vi "Blocking Performance Test Core.vi"(6 "Packets Sent":refnum<vi>, 8 "error in":errorcluster, 10 "test run":string="fbf_1", 11 "Test Paramaters":T1={"Interference sig. freq."=30, "Wanted Signal"=2426.0, "Blocking Signal"=2426.0, "Measurement res."=10} {"Measurement res." format="%.0f MHz"; "Blocking Signal" format="%#_gdBm"; "Interference sig. freq." format="%.0f MHz"; "Wanted Signal" format="%#_gdBm"}) -> (0 "error out":errorcluster, 1 "PER":dbl, 2 "Results":string, 3 "received Packets":u32)   [LabVIEW 2013]
doc: "This state machine will perform a single test based on a set of paramaters fed into the input and provide a set of results."
uses:
  Test Parameters.ctl
  Main Test Control.ctl
  Sig Gen Control Command.ctl
  Waveform Details Control.ctl
  UUT Control Command.ctl
  Globals/Hardware Configuration Global.vi
  Globals/Test Criteria Global.vi
panel:
  out "Send Packet Count":u32
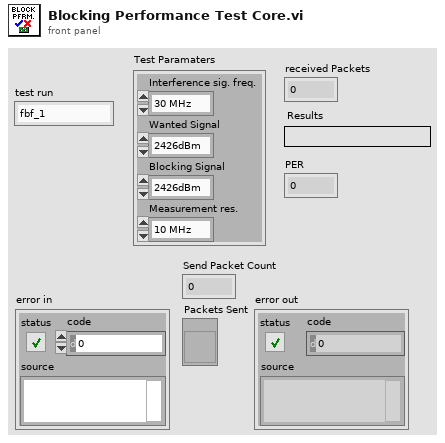
[diagram p1: front panel]
types:
  T1 = typedef "Test Parameters.ctl" = cluster{"Interference sig. freq.":u32, "Wanted Signal":dbl, "Blocking Signal":dbl, "Measurement res.":u32}
  T2 = typedef "Main Test Control.ctl" = enum16{"Initialise", "Stop", "Init WFG 1", "Init WFG 2", "Validate Temperature", "Init UUT", "Begin Test", "Send Packet", "Check Received Packets", "Temerature correction cycle"}
  T3 = typedef "Waveform Details Control.ctl" = cluster{"Power (dB)":dbl, "Frequency (MHz)":u32}
  T4 = typedef "Sig Gen Control Command.ctl" = enum16{"Initialise", "Start", "Stop", "Set Frequency", "Set Power", "Send Packet"}
  T5 = typedef "UUT Control Command.ctl" = enum16{"Initialise packet count", "Read Packet Count", "Return Temperature", "Return Operating Voltage"}
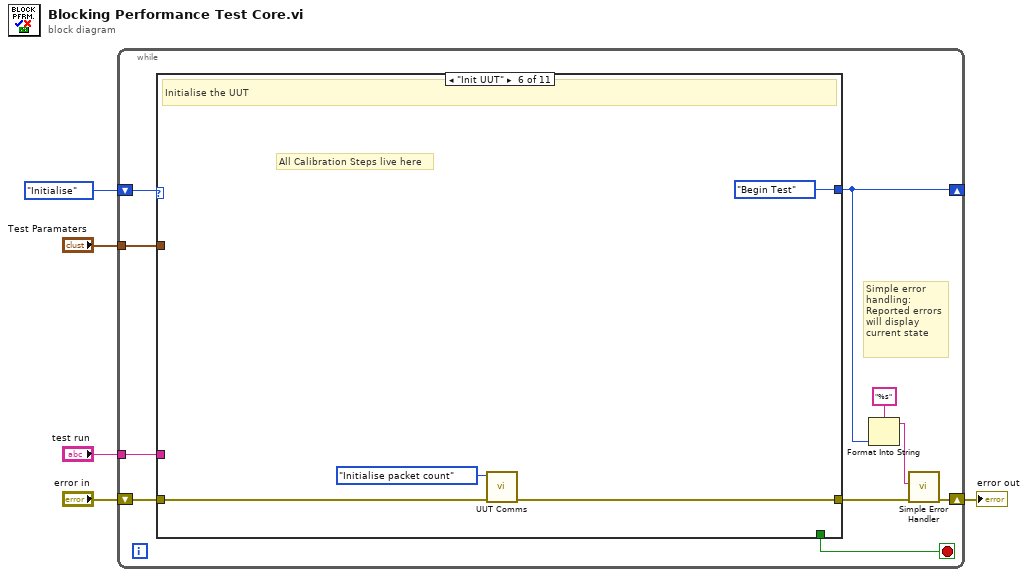
[diagram p0: block diagram]
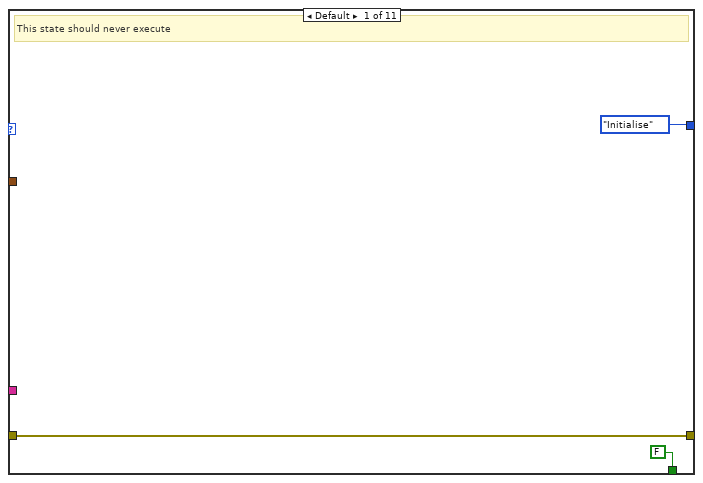
[diagram p2: hidden frame]
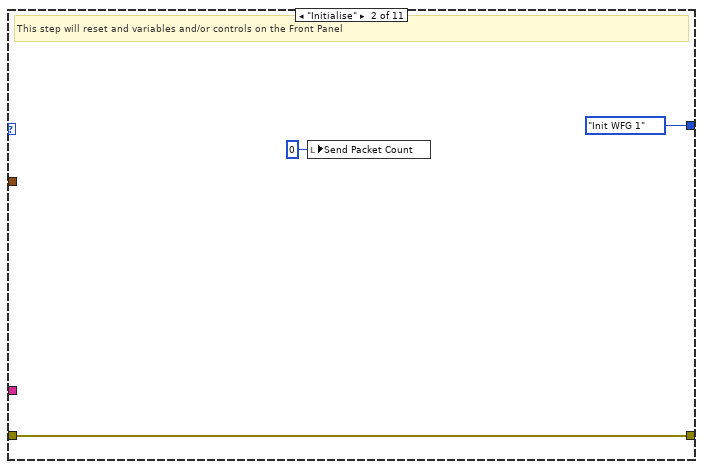
[diagram p3: hidden frame]
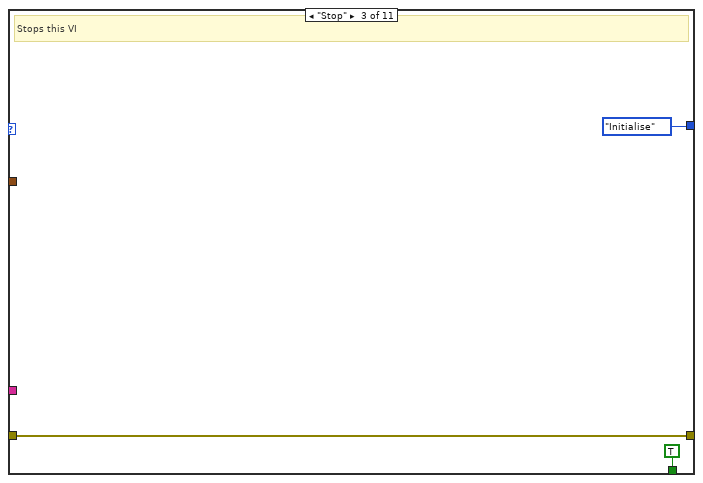
[diagram p4: hidden frame]
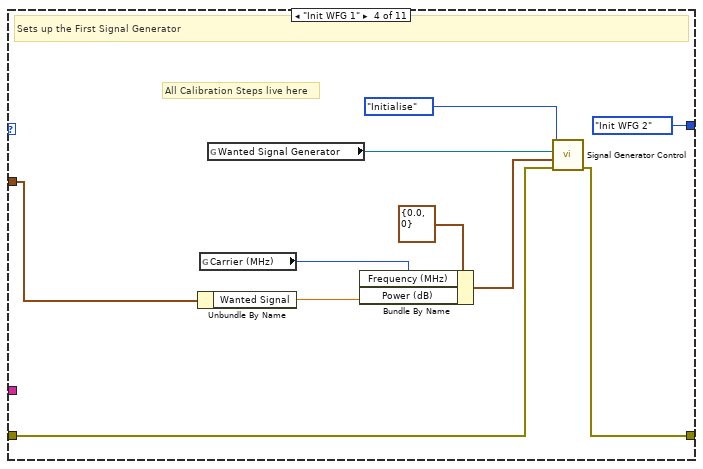
[diagram p5: hidden frame]
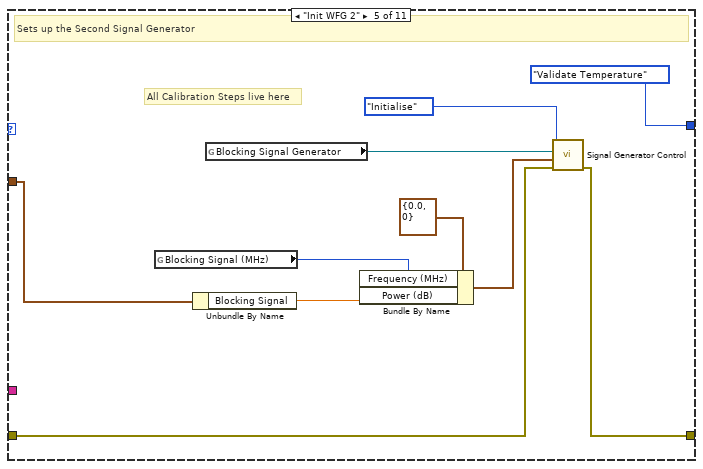
[diagram p6: hidden frame]
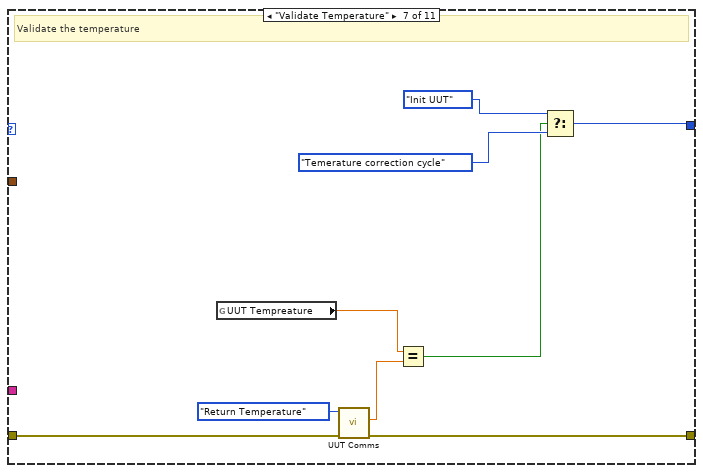
[diagram p7: hidden frame]
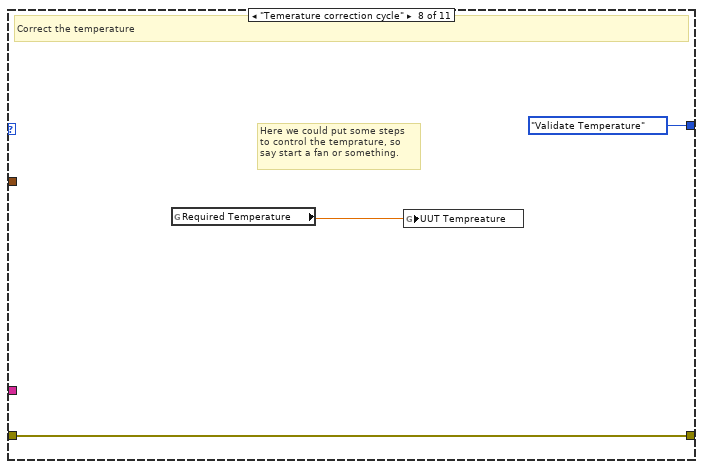
[diagram p8: hidden frame]
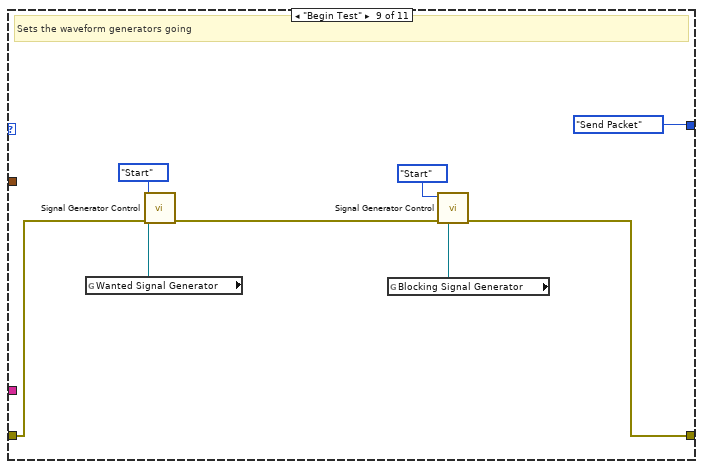
[diagram p9: hidden frame]
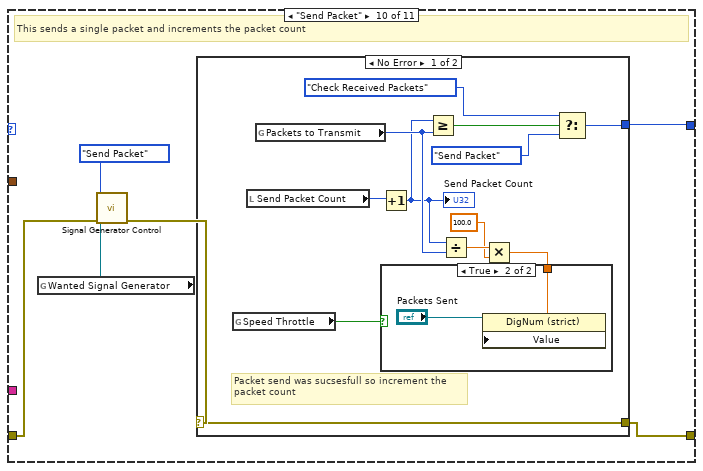
[diagram p10: hidden frame]
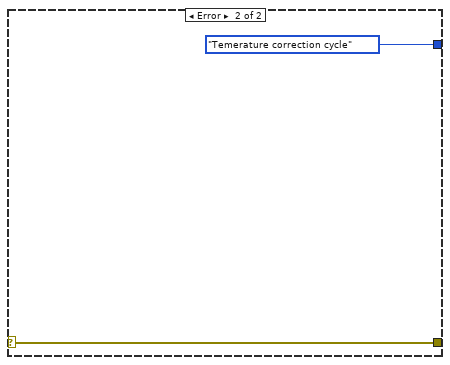
[diagram p12: hidden frame]
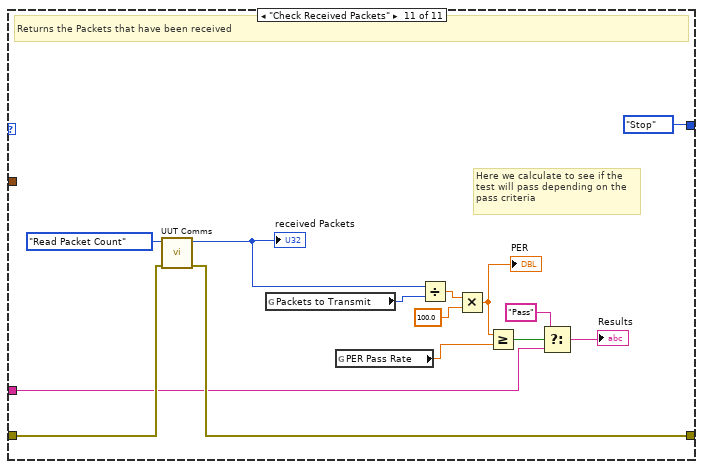
[diagram p13: hidden frame]
diagram:
  n1 = while {
    shift-right: [w10] -> _
    shift-left: Main_Test_Control."Initialise" ("Control") -> [w14]
    shift-right: [w11] -> w3
    shift-left: "error in" -> [w13]
    tunnel: "Test Paramaters" -> [w7]
    tunnel: "test run" -> [w6]
    stop <- w15 stop-if-true
    # "Simple error\nhandling:\nReported errors\nwill display\ncurrent state"
    n2 = case shown="\"Init UUT\"" w14 {
      tunnel: [FALSE _ TRUE _ _ _ _ _ _ _ _] -> w15
      tunnel: [Main_Test_Control."Initialise" ("Control") Main_Test_Control."Init WFG 1" ("Control") Main_Test_Control."Initialise" ("Control") Main_Test_Control."Init WFG 2" ("Control") Main_Test_Control."Validate Temperature" ("Control") Main_Test_Control."Begin Test" ("Control") w52 Main_Test_Control."Validate Temperature" ("Control") Main_Test_Control."Send Packet" ("Control") w69 Main_Test_Control."Stop" ("Control")] -> w10
      tunnel: w13 -> [w16 w19 w22 w29 w39 w48 w57 w59 w63 w72 w103]
      tunnel: [w16 w19 w22 w28 w38 w47 w56 w59 w62 w70 w102] -> w12
      tunnel: w7 -> [_ _ _ w26 w37 _ _ _ _ _ _]
      tunnel: w6 -> [_ _ _ _ _ _ _ _ _ _ w91]
      frame Default {
        # "This state should never execute"
      }
      frame "Initialise" {
        # "This step will reset and variables and/or controls on the Front Panel"
        n3 = local write "Send Packet Count"(u32 0 ("Send Packet Count")) -> ()
      }
      frame "Stop" {
        # "Stops this VI"
      }
      frame "Init WFG 1" {
        # "All Calibration Steps live here"
        # "Sets up the First Signal Generator"
        n4 = Unbundle By Name(w26) -> ("Wanted Signal"=w25:dbl)
        n5 = global read "Test Criteria Global.vi" "Carrier (MHz)"() -> (w27:u32)
        n6 = global read "Hardware Configuration Global.vi" "Wanted Signal Generator"() -> (w33:refnum<k15>)
        n7 = Bundle By Name(cluster=T3 {"Power (dB)"=0.0, "Frequency (MHz)"=0} ("Waveform Data"), "Frequency (MHz)"=w27, "Power (dB)"=w25) -> (w30:T3)
        n8 = call "Signal Generator Control.vi"("error in"=w29, "Waveform Data"=w30, "Device"=w33, "Command"=Sig_Gen_Control_Command."Initialise") -> ("error out"=w28:errorcluster)  [unwired: 6 in, 1 out]
      }
      frame "Init WFG 2" {
        # "All Calibration Steps live here"
        # "Sets up the Second Signal Generator"
        n9 = global read "Test Criteria Global.vi" "Blocking Signal (MHz)"() -> (w35:u32)
        n10 = Unbundle By Name(w37) -> ("Blocking Signal"=w36:dbl)
        n11 = global read "Hardware Configuration Global.vi" "Blocking Signal Generator"() -> (w43:refnum<k15>)
        n12 = Bundle By Name(cluster=T3 {"Power (dB)"=0.0, "Frequency (MHz)"=0} ("Waveform Data"), "Frequency (MHz)"=w35, "Power (dB)"=w36) -> (w40:T3)
        n13 = call "Signal Generator Control.vi"("error in"=w39, "Waveform Data"=w40, "Device"=w43, "Command"=Sig_Gen_Control_Command."Initialise") -> ("error out"=w38:errorcluster)  [unwired: 6 in, 1 out]
      }
      frame "Init UUT" {
        # "All Calibration Steps live here"
        # "Initialise the UUT"
        n14 = call "UUT Comms.vi"("error in"=w48, "Command"=UUT_Control_Command."Initialise packet count") -> ("error out"=w47:errorcluster)  [unwired: 6 in, 3 out]
      }
      frame "Validate Temperature" {
        # "Validate the temperature"
        n15 = global read "Test Criteria Global.vi" "UUT Tempreature"() -> (w51:dbl)
        n16 = call "UUT Comms.vi"("error in"=w57, "Command"=UUT_Control_Command."Return Temperature") -> ("error out"=w56:errorcluster, "Temperature"=w49:dbl)  [unwired: 6 in, 2 out]
        n17 = Equal?(x=w51, y=w49) -> (x = y?=w50:bool)
        n18 = Select(t=Main_Test_Control."Init UUT" ("Control"), s=w50, f=Main_Test_Control."Temerature correction cycle" ("Control")) -> (s? t:f=w52:T2)
      }
      frame "Temerature correction cycle" {
        # "Here we could put some steps\nto control the temprature, so\nsay start a fan or something."
        # "Correct the temperature"
        n19 = global read "Test Criteria Global.vi" "Required Temperature"() -> (w58:dbl)
        n20 = global write "Test Criteria Global.vi" "UUT Tempreature"(w58) -> ()
      }
      frame "Begin Test" {
        # "Sets the waveform generators going"
        n21 = global read "Hardware Configuration Global.vi" "Wanted Signal Generator"() -> (w68:refnum<k15>)
        n22 = call "Signal Generator Control.vi"("error in"=w63, "Device"=w68, "Command"=Sig_Gen_Control_Command."Start") -> ("error out"=w64:errorcluster)  [unwired: 7 in, 1 out]
        n23 = global read "Hardware Configuration Global.vi" "Blocking Signal Generator"() -> (w67:refnum<k15>)
        n24 = call "Signal Generator Control.vi"("error in"=w64, "Device"=w67, "Command"=Sig_Gen_Control_Command."Start") -> ("error out"=w62:errorcluster)  [unwired: 7 in, 1 out]
      }
      frame "Send Packet" {
        # "This sends a single packet and increments the packet count"
        n25 = global read "Hardware Configuration Global.vi" "Wanted Signal Generator"() -> (w74:refnum<k15>)
        n26 = call "Signal Generator Control.vi"("error in"=w72, "Device"=w74, "Command"=Sig_Gen_Control_Command."Send Packet") -> ("error out"=w71:errorcluster)  [unwired: 7 in, 1 out]
        n27 = case shown="No Error" w71 {
          selector: w71 -> [w81 w90]
          tunnel: [w81 w90] -> w70
          tunnel: [w82 Main_Test_Control."Temerature correction cycle" ("Control")] -> w69
          frame No Error {
            # "Packet send was sucsesfull so increment the\npacket count"
            n28 = global read "Test Criteria Global.vi" "Speed Throttle"() -> (w76:bool)
            n29 = local read "Send Packet Count"() -> (w86:u32)
            n30 = global read "Test Criteria Global.vi" "Packets to Transmit"() -> (w80:u32)
            n31 = Increment(x=w86) -> (x+1=w79:u32)
            "Send Packet Count" <- w79
            n32 = Greater Or Equal?(x=w79, y=w80) -> (x >= y?=w85:bool)
            n33 = Divide(x=w79, y=w80) -> (x/y=w78:dbl)
            n34 = Multiply(x=w78, y=100.0) -> (x*y=w77:dbl)
            n35 = case shown="True" w76 {
              tunnel: w77 -> [_ w87]
              frame False {
              }
              frame True {
                n36 = property class="DigNum (strict)"(reference="Packets Sent", "Value"=w87) -> ()  [unwired: 1 in, 2 out]
              }
            }
            n37 = Select(t=Main_Test_Control."Check Received Packets" ("Control"), s=w85, f=Main_Test_Control."Send Packet" ("Control")) -> (s? t:f=w82:T2)
          }
          frame Error {
          }
        }
      }
      frame "Check Received Packets" {
        # "Here we calculate to see if the\ntest will pass depending on the\npass criteria"
        # "Returns the Packets that have been received"
        n38 = call "UUT Comms.vi"("error in"=w103, "Command"=UUT_Control_Command."Read Packet Count") -> ("error out"=w102:errorcluster, "received Packets"=w100:u32)  [unwired: 6 in, 2 out]
        "received Packets" <- w100
        n39 = global read "Test Criteria Global.vi" "Packets to Transmit"() -> (w99:u32)
        n40 = global read "Test Criteria Global.vi" "PER Pass Rate"() -> (w95:dbl)
        n41 = Divide(x=w100, y=w99) -> (x/y=w98:dbl)
        n42 = Multiply(x=w98, y=100.0) -> (x*y=w96:dbl)
        "PER" <- w96
        n43 = Greater Or Equal?(x=w96, y=w95) -> (x >= y?=w94:bool)
        n44 = Select(t="Pass", s=w94, f=w91) -> (s? t:f=→"Results":string)
      }
    }
    n45 = Format Into String(format string="%s", w10) -> (resulting string=w9:string)  [unwired: 2 in, 1 out]
    n46 = call <vilib>:"Simple Error Handler.vi"("error source (\" \")"=w9, "error in (no error)"=w12) -> ("error out"=w11:errorcluster)  [unwired: 3 in, 4 out]
  }
  "error out" <- w3
